vi "verify error.vi"(8 "error in (no error)":errorcluster, 11 "Save Image in":refnum<class "Save Image.lvclass">) -> (0 "error out":errorcluster, 3 "Save Image out":refnum<class "Save Image.lvclass">)   [LabVIEW 2018, in "Save Image.lvclass"]
uses:
  Save Image.lvclass
  Save Image.lvclass/Save Image.ctl
  <vilib>/Utility/error.llb/Error Cluster From Error Code.vi
  <vilib>/ErrorRing/Error Ring.xnode
  Python Toolkit/Python Toolkit.lvclass
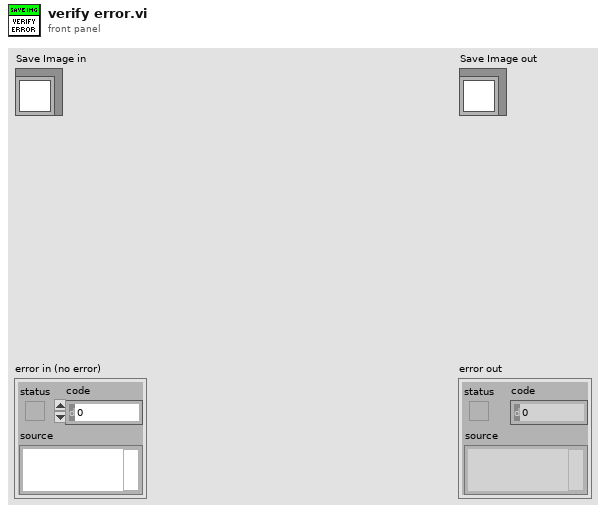
[diagram p1: front panel]
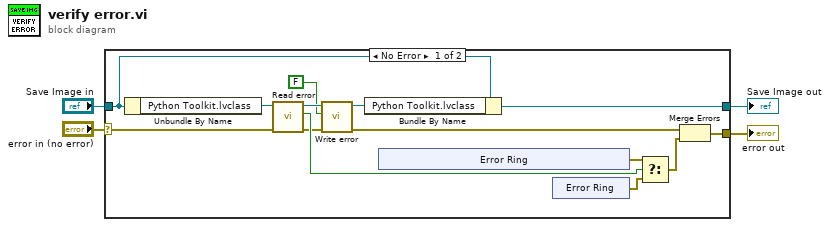
[diagram p0: block diagram]
diagram:
  n1 = case shown="No Error" "error in (no error)" {
    selector: "error in (no error)" -> [w14 w26]
    tunnel: [w12 w26] -> w3
    tunnel: [w8 w25] -> w1
    tunnel: "Save Image in" -> [w9 w25]
    frame No Error {
      n2 = Unbundle By Name(w9) -> ("Python Toolkit.lvclass"=w18:refnum<class "Python Toolkit.lvclass">)
      n3 = call-dynamic "Read error.vi"("error in (no error)"=w14, "Python Toolkit in"=w18) -> ("error out"=w11:errorcluster, "error"=w17:bool, "Python Toolkit out"=w6:refnum<class "Python Toolkit.lvclass">)  [unwired: 7 in]
      n4 = call-dynamic "Write error.vi"("error in (no error)"=w11, "error"=FALSE, "Python Toolkit in"=w6) -> ("error out"=w10:errorcluster, "Python Toolkit out"=w7:refnum<class "Python Toolkit.lvclass">)  [unwired: 7 in]
      n5 = Bundle By Name(cluster=w9, "Python Toolkit.lvclass"=w7) -> (w8:refnum<class "Save Image.lvclass">)
      n6 = xnode "Error Ring"() -> ("error out"=w16:errorcluster)
      n7 = xnode "Error Ring"() -> ("error out"=w15:errorcluster)
      n8 = Select(t=w16, s=w17, f=w15) -> (s? t:f=w13:errorcluster)
      n9 = Merge Errors(w10, w13) -> (w12:errorcluster)
    }
    frame Error {
    }
  }
  "error out" <- w3
  "Save Image out" <- w1
